vi "Run Framework Configuration.vi"() -> ()   [LabVIEW 2017]
uses:
  Classes/Framework/Framework Options.ctl
  Typedefs/DSF FIFO Options.ctl
  Classes/Thread/Thread Options.ctl
  Typedefs/DSF Plugin Options.ctl
  Typedefs/DSF Performance Options.ctl
  Typedefs/DSF Engine Framework Configuration.ctl
  Typedefs/DSF Engine Plugin Configuration.ctl
  Typedefs/DSF Timing Info.ctl
  Typedefs/DSF Engine Plugin Thread Configuration.ctl
  Typedefs/DSF Settings Info.ctl
  Typedefs/DSF Engine Transfer Group Configuration.ctl
  Typedefs/DSF Direction.ctl
  Typedefs/DSF Engine Transfer Configuration.ctl
  Typedefs/DSF Byte Order.ctl
  Typedefs/DSF Engine Channel Configuration.ctl
  Typedefs/DSF Data Type.ctl
  Typedefs/DSF Timeout Behavior.ctl
  Typedefs/DSF UI Pointers.ctl
  <vilib>/NI/Memory Manager/Classes/Pointer/Pointer.lvclass
  <vilib>/NI/Memory Manager/Classes/Pointer/Pointer.lvclass/Pointer.ctl
  <vilib>/NI/Memory Manager/Classes/Pointer/Write U32.vi
  <vilib>/NI/Memory Manager/Classes/Pointer/Read U32.vi
  <vilib>/NI/Memory Manager/Classes/Pointer/Read I32.vi
  <vilib>/NI/Memory Manager/Classes/Pointer/Read Bool.vi
  <vilib>/NI/Memory Manager/Classes/Pointer/Write Bool.vi
  <vilib>/NI/Memory Manager/Classes/Pointer/Set Address.vi
  <vilib>/NI/Memory Manager/Classes/Pointer/Set Size.vi
  <vilib>/NI/Memory Manager/Classes/Pointer/Set Internal.vi
  <vilib>/NI/Memory Manager/Classes/Pointer/Clear.vi
  <vilib>/NI/Memory Manager/Classes/Pointer/Write (No Check).vi
  <vilib>/NI/Memory Manager/Classes/Pointer/Write (No Check) U32.vi
  <vilib>/NI/Memory Manager/Classes/Pointer/Check Move.vi
  <vilib>/NI/Memory Manager/Classes/Pointer/Read (No Check).vi
  <vilib>/NI/Memory Manager/Classes/Pointer/Read (No Check) U32.vi
  <vilib>/NI/Memory Manager/Classes/Pointer/Read (No Check) I32.vi
  <vilib>/NI/Memory Manager/Classes/Pointer/Read (No Check) Bool.vi
  <vilib>/NI/Memory Manager/Classes/Pointer/Write (No Check) Bool.vi
  <vilib>/NI/Memory Manager/Classes/Pointer/Check Null Pointer.vi
  <vilib>/NI/Memory Manager/Classes/Pointer/Clear (No Check).vi
  <vilib>/NI/Memory Manager/Classes/Pointer/Check Length.vi
  <vilib>/NI/Memory Manager/Classes/Pointer/Get Address.vi
  <vilib>/NI/Memory Manager/Classes/Pointer/Check Count.vi
  <vilib>/NI/Memory Manager/Classes/Pointer/Check Bounds (Power of 2).vi
  <vilib>/NI/Memory Manager/Classes/Pointer/Errors.vi
  <vilib>/NI/Memory Manager/Classes/Pointer/Null Pointer.vi
  <vilib>/NI/Memory Manager/Classes/Pointer/Is Null.vi
  <vilib>/NI/Memory Manager/Classes/Pointer/Get Size.vi
  <vilib>/NI/Memory Manager/Classes/Pointer/Check Bounds (Pointer).vi
  <vilib>/NI/Memory Manager/Classes/Pointer/Out of Bounds.vi
  <vilib>/NI/Memory Manager/Classes/Pointer/Check Bounds.vi
  <vilib>/NI/Memory Manager/Classes/Pointer/Create Error.vi
  <vilib>/NI/Memory Manager/Classes/Pointer/Write Pointer Size to Error.vi
  <vilib>/NI/Memory Manager/Classes/Pointer/Check Bounds (Buffer).vi
  <vilib>/NI/Memory Manager/Constants/Constants.vi
  <vilib>/NI/Memory Manager/Constants/Library Name.vi
  <vilib>/NI/Memory Manager/Classes/Pointer/Pointer Error Info.vi
  <vilib>/NI/Memory Manager/Constants/Pointer Class Name.vi
  <vilib>/NI/Memory Manager/Classes/Pointer/Buffer Underflow.vi
  <vilib>/NI/Memory Manager/VIs/New Error Cluster.vi
  <vilib>/NI/Memory Manager/VIs/New Error Cluster (512B).vi
  <vilib>/NI/Memory Manager/VIs/Set Error Status.vi
  <vilib>/NI/Memory Manager/VIs/Set Error Code.vi
  <vilib>/NI/Memory Manager/VIs/Set Error Source.vi
  <vilib>/NI/Memory Manager/VIs/Write String to Source.vi
  <vilib>/NI/Memory Manager/VIs/Write Numeric to Source.vi
  <vilib>/NI/Memory Manager/VIs/Write Numeric Scalar to Source (Base10 U64).vi
  Classes/Configuration/Configuration Session.lvclass
  DSF Core.lvlib
  Classes/Framework/Framework.lvclass
  Classes/Thread/Thread.lvclass
panel:
  in  "thread settings":cluster{"Processor":i32, "Priority":i32}={"Processor"=-2, "Priority"=100}
  out "framework configuration":T1
  out "actual frequency":u32 format="%.0pHz"
  in  "target frequency":u32=100 format="%.0pHz"
  in  "components directory":path
  in  "dsf configuration file path":path=path "C:/Users/Admin/Desktop/test.dsf"
  out "iteration":i32
  out "error out":errorcluster
  in  "framework options":T13={"FIFO Options"={"Infinite Timeouts"=FALSE}, "Thread Options"={"Show FP On Call"=TRUE, "Close FP After Call"=TRUE, "Allow Debugging"=TRUE, "Restart On Error"=FALSE}, "Plugin Options"={"Default Components"=TRUE}, "Performance Options"={"Measure Period"=TRUE, "Measure Rx/Tx Duration"=TRUE}}
  in  "stop":bool
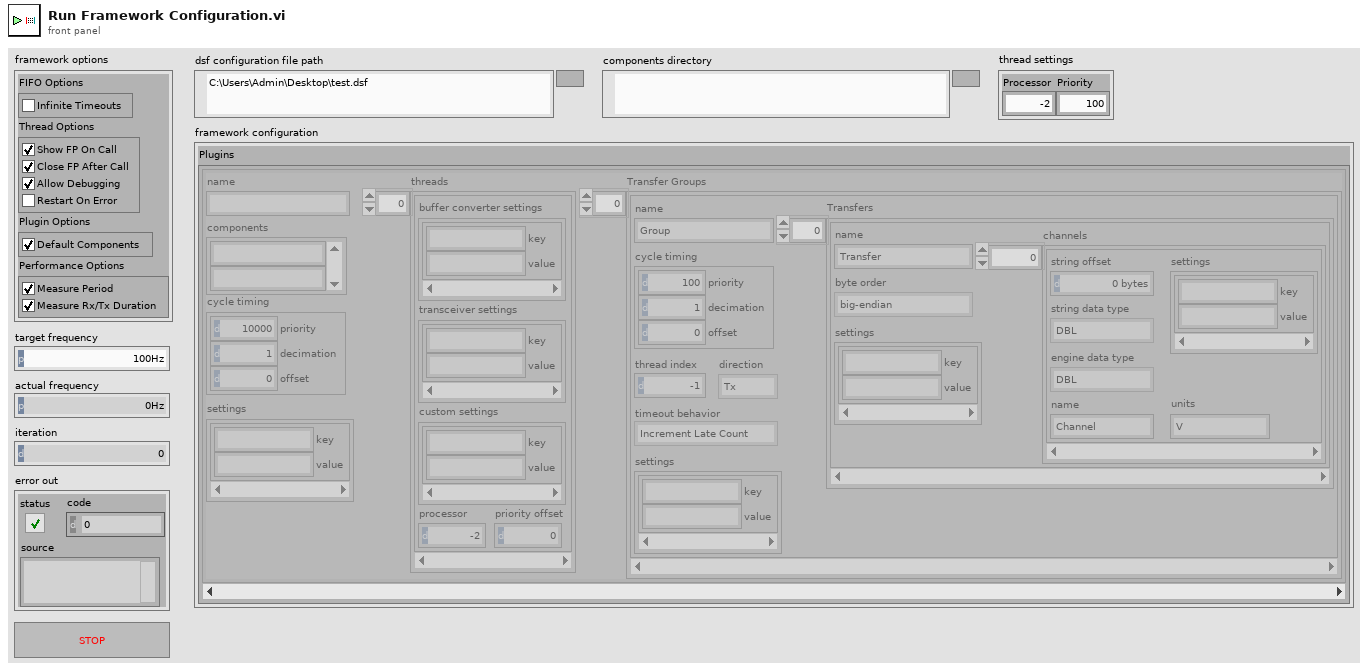
[diagram p1: front panel]
types:
  T1 = typedef "DSF Core.lvlib/DSF Engine Framework Configuration.ctl" = cluster{"Plugins":T2[]}
  T2 = typedef "DSF Core.lvlib/DSF Engine Plugin Configuration.ctl" = cluster{"name":string, "components":string[], "cycle timing":T3, "threads":T4[], "Transfer Groups":T6[], "settings":T5}
  T3 = typedef "DSF Core.lvlib/DSF Timing Info.ctl" = cluster{"priority":u64, "decimation":u64, "offset":u64}
  T4 = typedef "DSF Core.lvlib/DSF Engine Plugin Thread Configuration.ctl" = cluster{"buffer converter settings":T5, "transceiver settings":T5, "custom settings":T5, "processor":i32, "priority offset":i16}
  T5 = typedef "DSF Core.lvlib/DSF Settings Info.ctl" = cluster{"key":string, "value":string}[]
  T6 = typedef "DSF Core.lvlib/DSF Engine Transfer Group Configuration.ctl" = cluster{"name":string, "direction":T7, "cycle timing":T3, "thread index":i32, "settings":T5, "Transfers":T8[], "timeout behavior":T12}
  T7 = typedef "DSF Core.lvlib/DSF Direction.ctl" = enum8{"Tx", "Rx"}
  T8 = typedef "DSF Core.lvlib/DSF Engine Transfer Configuration.ctl" = cluster{"name":string, "byte order":T9, "settings":T5, "channels":T10[]}
  T9 = typedef "DSF Core.lvlib/DSF Byte Order.ctl" = enum8{"big-endian", "little-endian"}
  T10 = typedef "DSF Core.lvlib/DSF Engine Channel Configuration.ctl" = cluster{"string offset":u64, "string data type":T11, "engine data type":T11, "name":string, "settings":T5, "units":string}
  T11 = typedef "DSF Core.lvlib/DSF Data Type.ctl" = enum8{"Bool", "SGL", "DBL", "I8", "I16", "I32", "I64", "U8", "U16", "U32", "U64"}
  T12 = typedef "DSF Core.lvlib/DSF Timeout Behavior.ctl" = enum8{"Increment Late Count", "Throw Error"}
  T13 = typedef "DSF Core.lvlib/Framework.lvclass/Framework Options.ctl" = cluster{"FIFO Options":T14, "Thread Options":T15, "Plugin Options":T16, "Performance Options":T17}
  T14 = typedef "DSF Core.lvlib/Framework.lvclass/DSF FIFO Options.ctl" = cluster{"Infinite Timeouts":bool}
  T15 = typedef "DSF Core.lvlib/Thread.lvclass/Thread Options.ctl" = cluster{"Show FP On Call":bool, "Close FP After Call":bool, "Allow Debugging":bool, "Restart On Error":bool}
  T16 = typedef "DSF Core.lvlib/Framework.lvclass/DSF Plugin Options.ctl" = cluster{"Default Components":bool}
  T17 = typedef "DSF Core.lvlib/DSF Performance Options.ctl" = cluster{"Measure Period":bool, "Measure Rx/Tx Duration":bool}
  T18 = typedef "DSF Core.lvlib/DSF UI Pointers.ctl" = cluster{"Stop":refnum<class "Pointer.lvclass">, "Target Period":refnum<class "Pointer.lvclass">, "Actual Period":refnum<class "Pointer.lvclass">, "Iteration":refnum<class "Pointer.lvclass">}
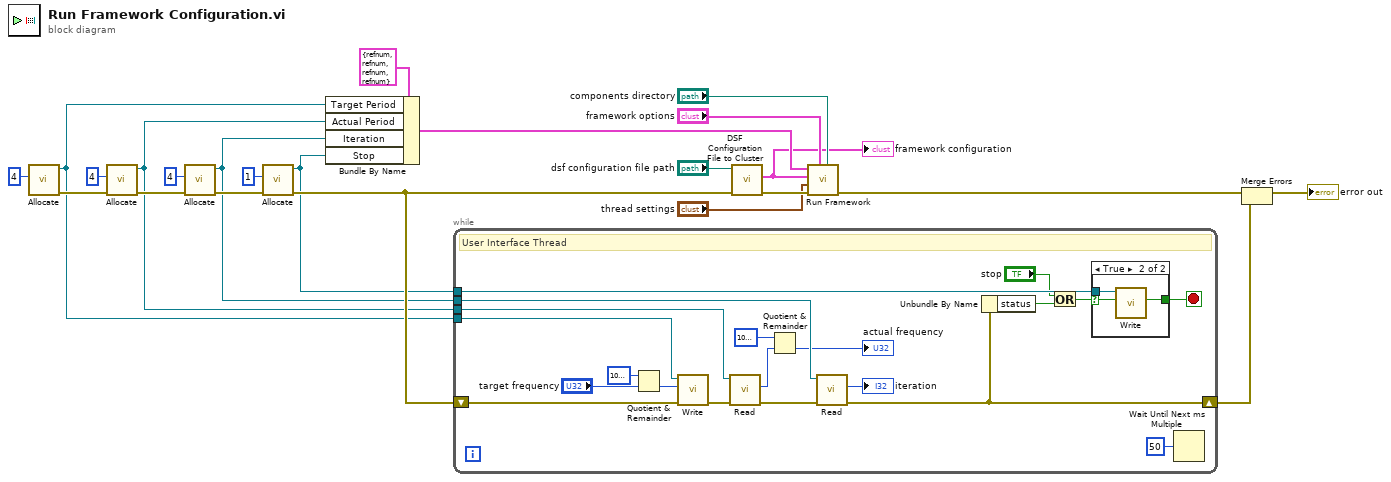
[diagram p0: block diagram]
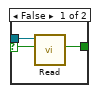
[diagram p2: hidden frame]
diagram:
  n1 = call <vilib>:"Allocate.vi"("size"=u64 4) -> ("error out"=w16:errorcluster, "Pointer out"=w8:refnum<class "Pointer.lvclass">)  [unwired: 9 in]
  n2 = call <vilib>:"Allocate.vi"("error in (no error)"=w16, "size"=u64 4) -> ("error out"=w18:errorcluster, "Pointer out"=w9:refnum<class "Pointer.lvclass">)  [unwired: 8 in]
  n3 = call <vilib>:"Allocate.vi"("error in (no error)"=w18, "size"=u64 4) -> ("error out"=w13:errorcluster, "Pointer out"=w10:refnum<class "Pointer.lvclass">)  [unwired: 8 in]
  n4 = call <vilib>:"Allocate.vi"("error in (no error)"=w13, "size"=u64 1) -> ("error out"=w23:errorcluster, "Pointer out"=w6:refnum<class "Pointer.lvclass">)  [unwired: 8 in]
  n5 = Bundle By Name(cluster=T18 {"Stop"=refnum, "Target Period"=refnum, "Actual Period"=refnum, "Iteration"=refnum} ("user interface pointers (null)"), "Target Period"=w8, "Actual Period"=w9, "Iteration"=w10, "Stop"=w6) -> (w2:T18)
  n6 = while {
    tunnel: w6 -> [w43]
    shift-right: [w32] -> w11
    shift-left: w23 -> [w39]
    tunnel: w8 -> [w36]
    tunnel: w9 -> [w34]
    tunnel: w10 -> [w31]
    stop <- w42 stop-if-true
    # "User Interface Thread"
    n7 = Quotient & Remainder(x=u32 1000000 ("y"), y="target frequency") -> (floor(x/y)=w35:u32)  [unwired: 1 out]
    n8 = call-poly <vilib>:"Write.vi"("error in (no error)"=w39, "value"=w35, "Pointer in"=w36) -> ("error out"=w37:errorcluster)  [unwired: 5 in, 3 out]
    n9 = call-poly <vilib>:"Read.vi"("error in (no error)"=w37, "Pointer in"=w34) -> ("error out"=w33:errorcluster, "value out"=w28:u32)  [unwired: 6 in, 2 out]
    n10 = Quotient & Remainder(x=u32 1000000 ("y"), y=w28) -> (floor(x/y)=→"actual frequency":u32)  [unwired: 1 out]
    n11 = call-poly <vilib>:"Read.vi"("error in (no error)"=w33, "Pointer in"=w31) -> ("error out"=w32:errorcluster, "value out"=→"iteration":i32)  [unwired: 6 in, 2 out]
    n12 = Unbundle By Name(w32) -> ("status"=w40:bool)
    n13 = Or(x="stop", y=w40) -> (x .or. y?=w41:bool)
    n14 = case shown="True" w41 {
      selector: w41 -> [w45 w48]
      tunnel: w43 -> [w46 w49]
      tunnel: [w44 w47] -> w42
      frame False {
        n15 = call-poly <vilib>:"Read.vi"("value in"=w45, "Pointer in"=w46) -> ("value out"=w44:bool)  [unwired: 6 in, 3 out]
      }
      frame True {
        n16 = call-poly <vilib>:"Write.vi"("value"=w48, "Pointer in"=w49) -> ("value"=w47:bool)  [unwired: 6 in, 3 out]
      }
    }
    n17 = Wait Until Next ms Multiple(millisecond multiple=u32 50) -> ()  [unwired: 1 out]
  }
  n18 = call "DSF Configuration File to Cluster.vi"("error in (no error)"=w23, "dsf configuration file path"="dsf configuration file path") -> ("error out"=w7:errorcluster, "framework configuration out"=w1:T1)  [unwired: 7 in, 1 out]
  "framework configuration" <- w1
  n19 = call "Run Framework.vi"("components directory"="components directory", "framework options"="framework options", "error in (no error)"=w7, "thread settings"="thread settings", "framework configuration"=w1, "user interface pointers (null)"=w2) -> ("error out"=w15:errorcluster)  [unwired: 5 in]
  n20 = Merge Errors(w15, w11) -> (→"error out":errorcluster)
